vi "Kalman_Filter_inner.vi"() -> ()   [LabVIEW 2020]
uses:
  <vilib>/Analysis/Matrix/Datatypes/RealMatrix.ctl
  <vilib>/Analysis/Matrix/NI_Matrix.lvlib
panel:
  in  "Accelerometer ANGLE in degrees":dbl format="%#_13g"
  in  "Gyro Velocity":dbl format="%#_13g"
  in  "Steady State Kalman Predictor Gain matrix":T1
  in  "F  Matrix":T1
  in  "H Matrix":T1
  out "X^ to register":dbl[](array[numeric])
  in  "X from register":dbl[](array[numeric])
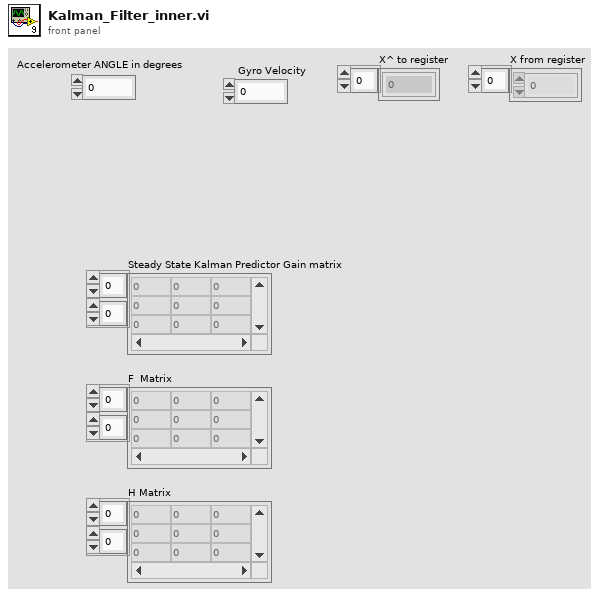
[diagram p1: front panel]
types:
  T1 = typedef "NI_Matrix.lvlib/RealMatrix.ctl" = dbl[][]
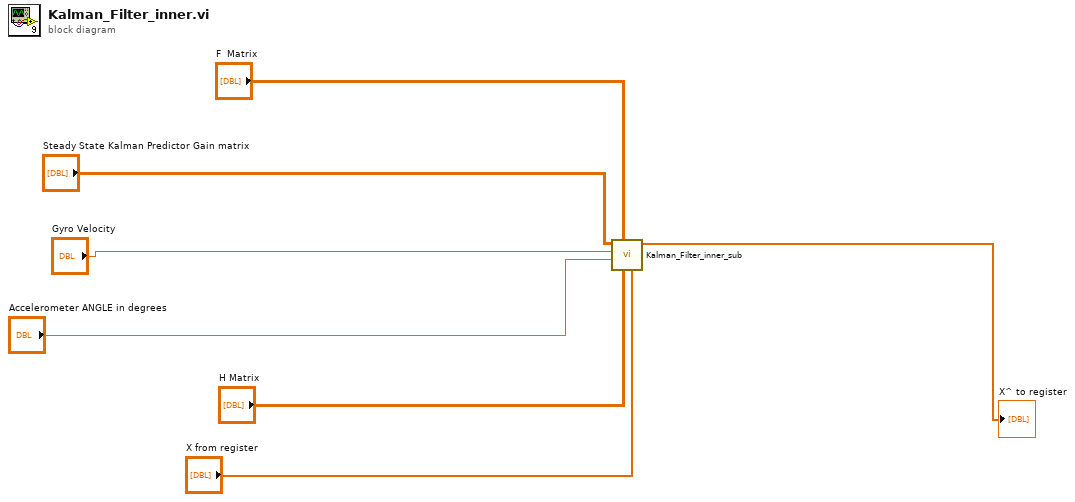
[diagram p0: block diagram]
diagram:
  n1 = call "Kalman_Filter_inner_sub.vi"("X from register"="X from register", "H Matrix"="H Matrix", "F  Matrix"="F  Matrix", "Accelerometer ANGLE in degrees"="Accelerometer ANGLE in degrees", "Gyro Velocity"="Gyro Velocity", "Steady State Kalman Predictor Gain matrix"="Steady State Kalman Predictor Gain matrix") -> ("X^ to register"=→"X^ to register":dbl[])  [unwired: 5 in]
